vi "Write_Results_file_with_Merge.vi"(3 "Values In":string[][](array[string]), 4 "Channel Names in":string[](array[string]), 5 "Filename":path) -> (0 "Values Out":string[][](array[string]), 1 "Channels Names Out":string[](array[string]))   [LabVIEW 2021]
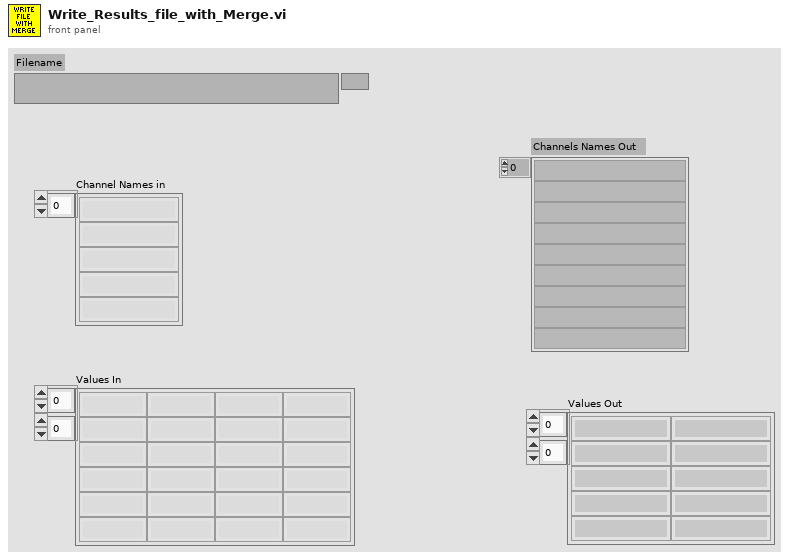
[diagram p1: front panel]
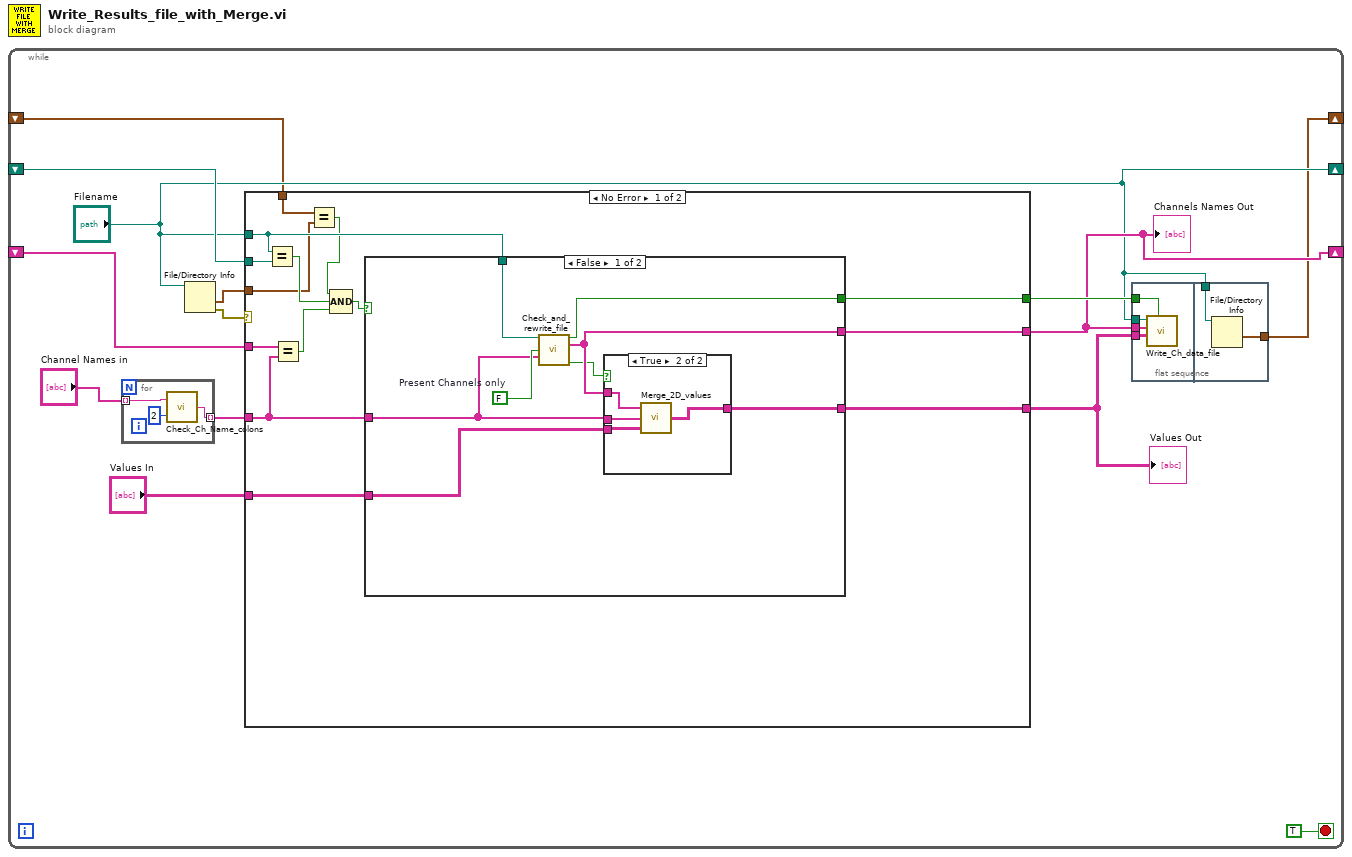
[diagram p0: block diagram]
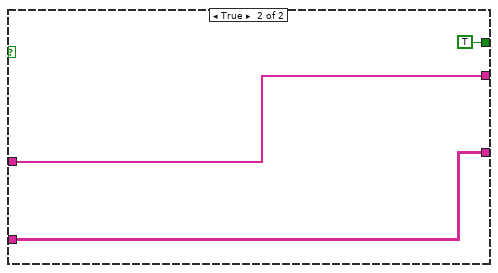
[diagram p3: hidden frame]
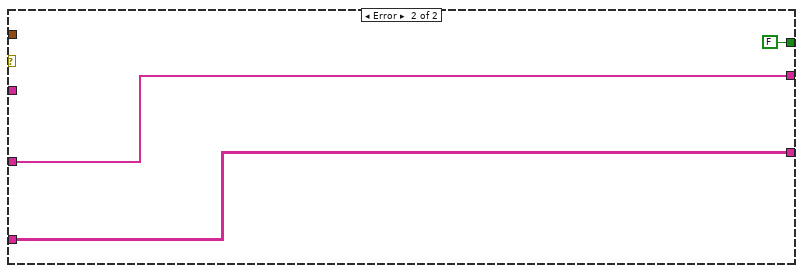
[diagram p4: hidden frame]
diagram:
  n1 = while {
    shift-right: [w10] -> _
    shift-left: _ -> [w8]
    shift-right: ["Filename"] -> _
    shift-left: _ -> [w9]
    shift-right: [w5] -> _
    shift-left: _ -> [w4]
    stop <- TRUE stop-if-true
    n2 = for {
      tunnel: "Channel Names in" -> [w17] mode=indexing
      tunnel: [w15] -> w1 mode=indexing
      n3 = call "Check_Ch_Name_colons.vi"("No of Colons"=2, "Ch Name in"=w17) -> ("Ch Name out"=w15:string)
    }
    n4 = File/Directory Info(path="Filename") -> (last mod=w3:timestamp, error out=w7:errorcluster)  [unwired: 1 in, 5 out]
    n5 = case shown="No Error" w7 {
      tunnel: [w37 w56] -> w10
      tunnel: [w36 w55] -> w14
      tunnel: w1 -> [w30 w56]
      tunnel: "Values In" -> [w35 w55]
      tunnel: [w34 FALSE ("exists?")] -> w12
      tunnel: "Filename" -> [w33 _]
      tunnel: w9 -> [w32 _]
      tunnel: w8 -> [w31 _]
      tunnel: w4 -> [w27 _]
      tunnel: w3 -> [w26 _]
      frame No Error {
        n6 = Equal?(x=w33, y=w32) -> (x = y?=w28:bool)
        n7 = Equal?(x=w31, y=w30) -> (x = y?=w29:bool)
        n8 = Equal?(x=w27, y=w26) -> (x = y?=w25:bool)
        n9 = Compound Arithmetic op=AND(w25, w28, w29) -> (w24:bool)
        n10 = case shown="False" w24 {
          tunnel: [w45 w52] -> w37
          tunnel: [w42 w51] -> w36
          tunnel: w35 -> [w41 w51]
          tunnel: [w40 TRUE ("exists?")] -> w34
          tunnel: w33 -> [w39 _]
          tunnel: w30 -> [w38 w52]
          frame False {
            w44 = FALSE  # Present Channels only
            n11 = call "Check_and_rewrite_file.vi"("Filename"=w39, "Present Channels only"=w44, "Present Channels"=w38) -> ("exists?"=w40:bool, "Merged Channels"=w45:string[], "Merged?"=w43:bool)  [unwired: 1 in, 9 out]
            n12 = case shown="True" w43 {
              tunnel: w41 -> [w46 w48]
              tunnel: w38 -> [_ w49]
              tunnel: [w46 w47] -> w42
              tunnel: w45 -> [_ w50]
              frame False {
              }
              frame True {
                n13 = call "Merge_2D_values.vi"("Values In"=w48, "Present Channels"=w49, "Desired Channels"=w50) -> ("Values Out"=w47:string[][])
              }
            }
          }
          frame True {
          }
        }
      }
      frame Error {
      }
    }
    "Values Out" <- w14
    "Channels Names Out" <- w10
    n14 = flat-sequence {
      tunnel: w14 -> [w21]
      tunnel: w12 -> [w20]
      tunnel: w10 -> [w19]
      tunnel: "Filename" -> [w18]
      tunnel: "Filename" -> [w23]
      tunnel: [w22] -> w5
      frame #0 {
        n15 = call "Write_Ch_data_file.vi"("exists?"=w20, "Channel Values"=w21, "Channel names"=w19, "Filename"=w18) -> ()  [unwired: 4 in, 4 out]
      }
      frame #1 {
        n16 = File/Directory Info(path=w23) -> (last mod=w22:timestamp)  [unwired: 1 in, 6 out]
      }
    }
  }
